vi "Lectura.vi"() -> ()   [LabVIEW 2020]
uses:
  <vilib>/Instr/_visa.llb/VISA Configure Serial Port (Instr).vi
panel:
  in  "stop":bool
  out "String 3":string
  in  "String 2":string
  in  "Boolean 2":bool
  out "String":string
  in  "Boolean":bool
  in  "VISA resource name":refnum<visa-resource-name>
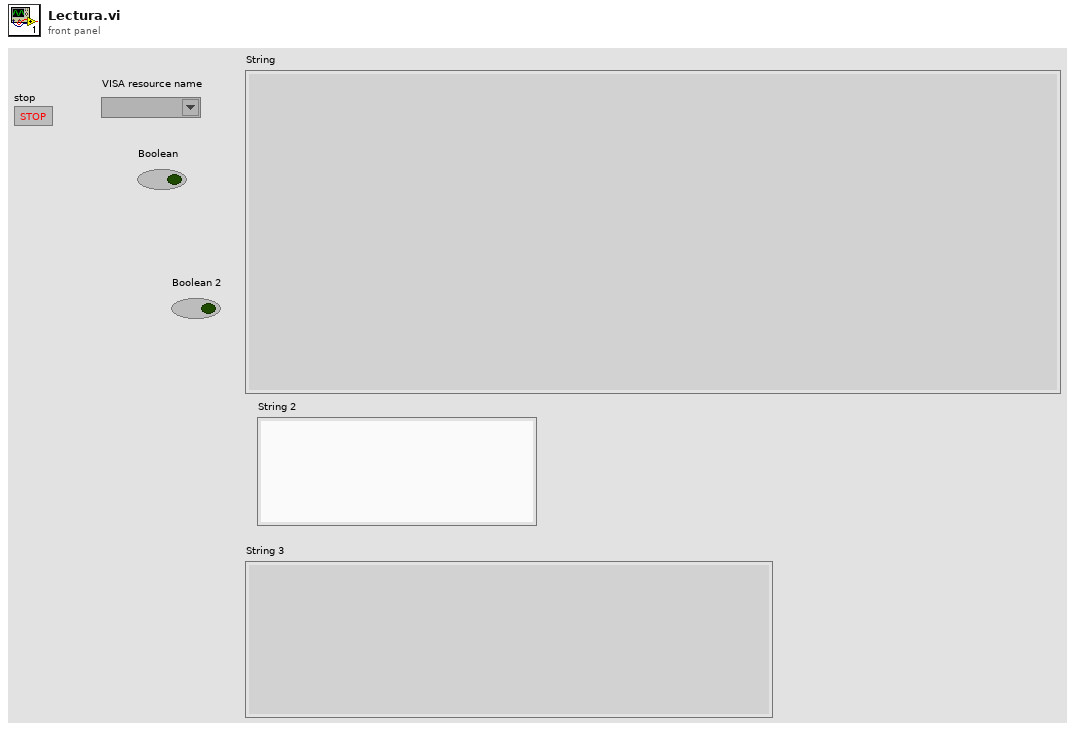
[diagram p1: front panel]
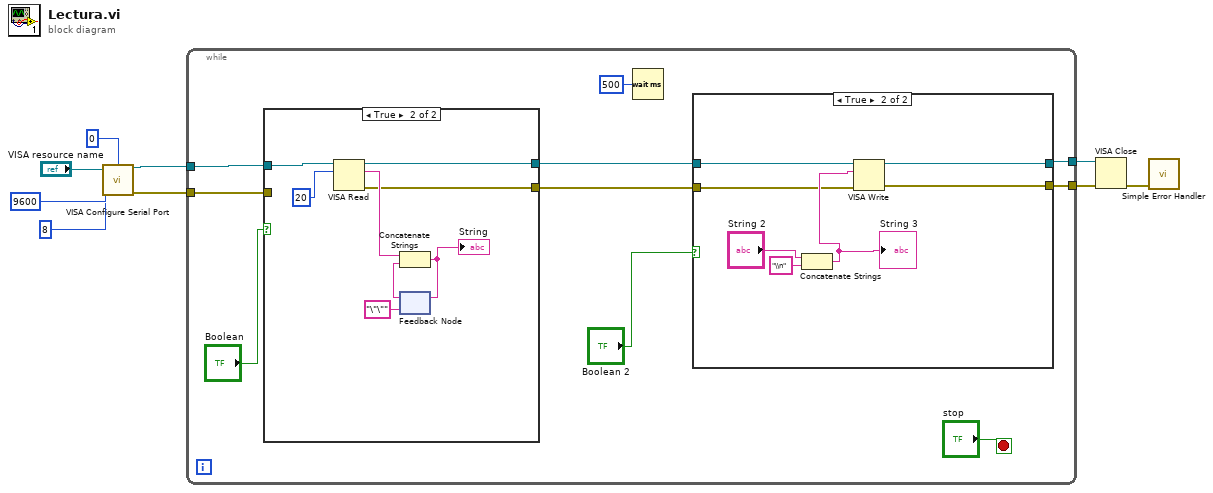
[diagram p0: block diagram]
diagram:
  n1 = call-poly "VISA Configure Serial Port"("VISA resource name"="VISA resource name", "termination char\n(0xA = '\\n' = LF)"=u8 0 ("termination char\n(0xA = '\\n' = LF)"), "baud rate (9600)"=u32 9600, "data bits (8)"=u16 8) -> ("VISA resource name out"=w5:refnum<visa-resource-name>, "error out"=w4:errorcluster)  [unwired: 10 in]
  n2 = while {
    tunnel: w5 -> [w17]
    tunnel: w4 -> [w16]
    tunnel: [w11] -> w3
    tunnel: [w10] -> w2
    stop <- "stop" stop-if-true
    n3 = case shown="True" "Boolean" {
      tunnel: w17 -> [w30 w38]
      tunnel: w16 -> [w29 _]
      tunnel: [w29 w32] -> w13
      tunnel: [w30 w31] -> w15
      frame False {
      }
      frame True {
        n4 = VISA Read(VISA resource name=w38, byte count=u32 20) -> (VISA resource name out=w31:refnum<visa-resource-name>, read buffer=w36:string, error out=w32:errorcluster)  [unwired: 1 in, 1 out]
        n5 = feedback #1("\"\"") -> (w34:string)
        n6 = Concatenate Strings(w36, w34) -> (w35:string)
        "String" <- w35
        n7 = feedback-in #1(w35) -> ()
      }
    }
    n8 = Wait (ms)(milliseconds to wait=u32 500) -> ()  [unwired: 1 out]
    n9 = case shown="True" "Boolean 2" {
      tunnel: w15 -> [w21 w28]
      tunnel: [w21 w27] -> w11
      tunnel: w13 -> [w20 w23]
      tunnel: [w20 w22] -> w10
      frame False {
      }
      frame True {
        n10 = Concatenate Strings("String 2", "\\n" ("string")) -> (w24:string)
        "String 3" <- w24
        n11 = VISA Write(VISA resource name=w28, write buffer=w24, error in (no error)=w23) -> (VISA resource name out=w27:refnum<visa-resource-name>, error out=w22:errorcluster)  [unwired: 1 out]
      }
    }
  }
  n12 = VISA Close(VISA resource name=w3, error in (no error)=w2) -> (error out=w1:errorcluster)
  n13 = call <vilib>:"Simple Error Handler.vi"("error in (no error)"=w1) -> ()  [unwired: 4 in, 5 out]
